vi "set_master_file.vi"(8 "error in (no error)":errorcluster, 11 "master file path":string) -> (0 "error out":errorcluster, 3 "master file path":path)   [LabVIEW 2017, in "worker.lvlib"]
uses:
  worker.lvlib
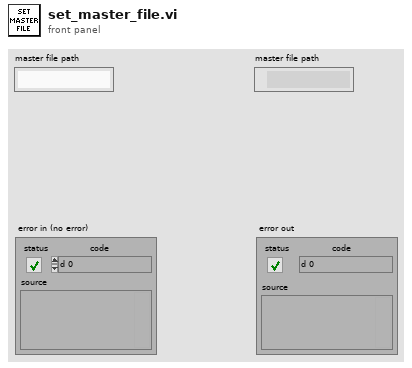
[diagram p1: front panel]
types:
  T1 = enum32{"invalid OS target", "Mac OS", "Windows 3.1", "Windows 95/NT", "Solaris 1", "Solaris 2", "HP-UX", "PowerMAX", "Linux", "Irix", "Rhapsody", "BeOS", "AIX", "OSF1", "VxWorks", "PharLap", "Carbon", "RTX", "Windows x64", "Linux x64", "Mac OS X x64"}
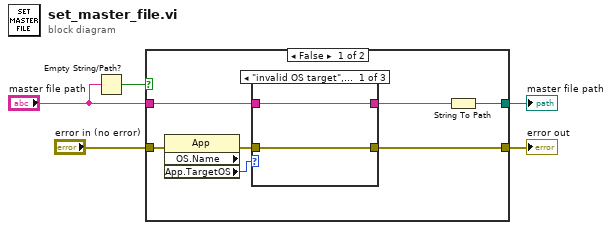
[diagram p0: block diagram]
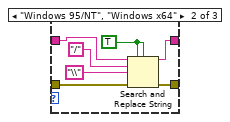
[diagram p2: hidden frame]
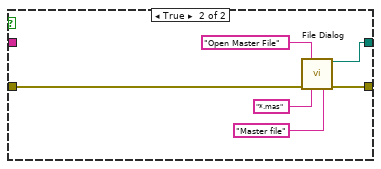
[diagram p4: hidden frame]
diagram:
  n1 = Empty String/Path?(string/path="master file path") -> (empty?=w5:bool)
  n2 = case shown="False" w5 {
    tunnel: [w7 w28] -> w3
    tunnel: "master file path" -> [w11 _]
    tunnel: "error in (no error)" -> [w10 w25]
    tunnel: [w8 w24] -> w1
    frame False {
      n3 = property class="App" props=["OS.Name", "App.TargetOS"](error in=w10) -> (error out=w9:errorcluster, "App.TargetOS"=w12:T1)  [unwired: 1 in, 2 out]
      n4 = case shown="\"invalid OS target\", Default" w12 {
        tunnel: w11 -> [w14 w18 w23]
        tunnel: w9 -> [w13 w17 w22]
        tunnel: [w13 w16 w22] -> w8
        tunnel: [w14 w15 w23] -> w6
        frame "invalid OS target", Default {
        }
        frame "Windows 95/NT", "Windows x64" {
          w21 = TRUE ("replace all? (F)")
          n5 = Search and Replace String(replace all?=w21, case sensitive?=w21, input string=w18, search string="/", replace string="\\" ("replace string (\"\")"), error in=w17) -> (result string=w15:string, error out=w16:errorcluster)  [unwired: 2 in, 2 out]
        }
        frame "Linux", "Linux x64" {
        }
      }
      n6 = String To Path(string=w6) -> (path=w7:path)
    }
    frame True {
      n7 = call "File Dialog"("prompt"="Open Master File", "error in"=w25, "pattern (all files)"="*.mas", "pattern label"="Master file") -> ("selected path"=w28:path, "error out"=w24:errorcluster)  [unwired: 8 in, 2 out]
    }
  }
  "error out" <- w1
  "master file path" <- w3
